vi "toString.vi"(7 "UTC? (F)":bool, 9 "Timestamp (now)":timestamp, 11 "DateTime.ISO8601 in":refnum<class "DateTime.ISO8601.lvclass">) -> (1 "DateTime String":string, 3 "DateTime.ISO8601 out":refnum<class "DateTime.ISO8601.lvclass">)   [LabVIEW 2013, in "DateTime.ISO8601.lvclass"]
uses:
  DateTime.ISO8601.lvclass
  DateTime.ISO8601.lvclass/DateTime.ISO8601.ctl
  Timestamp to ISO8601 Day.vi
  isLeapYear (timestamp).vi
  Timestamp to ISO8601 Year.vi
  isLeapYear (integer).vi
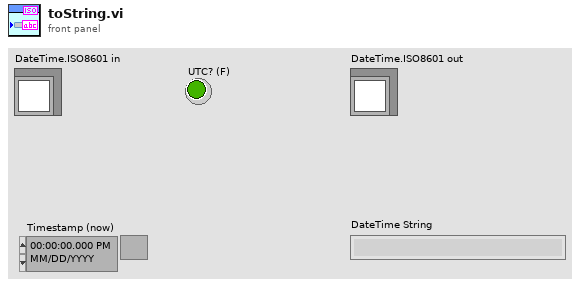
[diagram p1: front panel]
types:
  T1 = typedef "ISO8601 Date Formats.ctl" = enum16{"UTC Date-Time", "ISO Time", "Date", "Calendar Month", "Week", "Week-Day", "Month-Day", "Ordinal Date"}
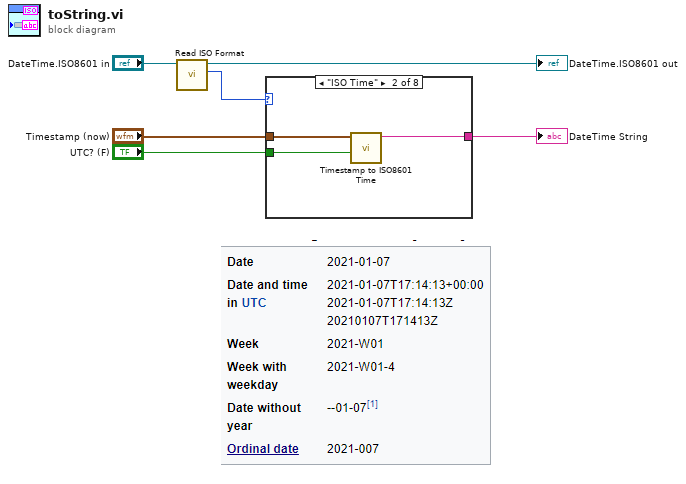
[diagram p0: block diagram]
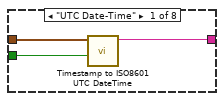
[diagram p2: hidden frame]
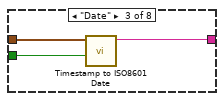
[diagram p3: hidden frame]
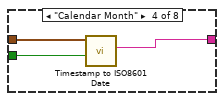
[diagram p4: hidden frame]
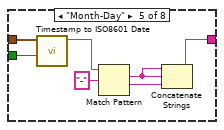
[diagram p5: hidden frame]
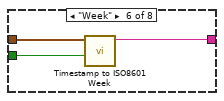
[diagram p6: hidden frame]
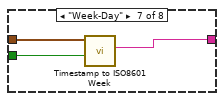
[diagram p7: hidden frame]
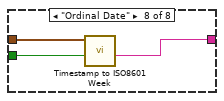
[diagram p8: hidden frame]
diagram:
  n1 = call "Read ISO Format.vi"("DateTime.ISO8601 in"="DateTime.ISO8601 in") -> ("ISO Format"=w1:T1, "DateTime.ISO8601 out"=→"DateTime.ISO8601 out":refnum<class "DateTime.ISO8601.lvclass">)  [unwired: 9 in]
  n2 = case shown="\"ISO Time\"" w1 {
    tunnel: "Timestamp (now)" -> [w9 w12 w15 w18 w25 w28 w31 w34]
    tunnel: [w8 w10 w13 w16 w20 w26 w29 w32] -> w5
    tunnel: "UTC? (F)" -> [w7 w11 w14 w17 w24 w27 w30 w33]
    frame "UTC Date-Time" {
      n3 = call "Timestamp to ISO8601 UTC DateTime.vi"("UTC? (F)"=w7, "Timestamp (now)"=w9) -> ("ISO8601 UTC DateTime"=w8:string)  [unwired: 9 in]
    }
    frame "ISO Time" {
      n4 = call "Timestamp to ISO8601 Time.vi"("UTC? (F)"=w11, "Timestamp (now)"=w12) -> ("ISO8601 Time"=w10:string)  [unwired: 9 in]
    }
    frame "Date" {
      n5 = call "Timestamp to ISO8601 Date.vi"("UTC? (F)"=w14, "Timestamp (now)"=w15) -> ("ISO8601 Date"=w13:string)  [unwired: 8 in, 1 out]
    }
    frame "Calendar Month" {
      n6 = call "Timestamp to ISO8601 Date.vi"("UTC? (F)"=w17, "Timestamp (now)"=w18) -> ("ISO8601 Calendar Month"=w16:string)  [unwired: 8 in, 1 out]
    }
    frame "Month-Day" {
      n7 = call "Timestamp to ISO8601 Date.vi"("UTC? (F)"=w24, "Timestamp (now)"=w25) -> ("ISO8601 Date"=w21:string)  [unwired: 8 in, 1 out]
      n8 = Match Pattern(string=w21, regular expression="-") -> (match substring=w19:string, after substring=w22:string)  [unwired: 1 in, 2 out]
      n9 = Concatenate Strings(w19, w19, w22) -> (w20:string)
    }
    frame "Week" {
      n10 = call "Timestamp to ISO8601 Week.vi"("UTC? (F)"=w27, "Timestamp (now)"=w28) -> ("ISO8601 Week"=w26:string)  [unwired: 7 in, 2 out]
    }
    frame "Week-Day" {
      n11 = call "Timestamp to ISO8601 Week.vi"("UTC? (F)"=w30, "Timestamp (now)"=w31) -> ("ISO8601 Weekday"=w29:string)  [unwired: 7 in, 2 out]
    }
    frame "Ordinal Date" {
      n12 = call "Timestamp to ISO8601 Week.vi"("UTC? (F)"=w33, "Timestamp (now)"=w34) -> ("ISO8601 Ordinal Date"=w32:string)  [unwired: 7 in, 2 out]
    }
  }
  "DateTime String" <- w5
